vi "LeftClick.vi"(6 "Double Click":bool, 7 "Table History ref":refnum<vi>, 8 "error in (no error)":errorcluster, 9 "Table CtlRef In":refnum<vi>, 10 "Cell Position":T1, 11 "ModeCol in":refnum<class "ModeCol.lvclass">) -> (0 "error out":errorcluster, 1 "Table CtlRef Out":refnum<vi>, 2 "Discard?":bool, 3 "ModeCol out":refnum<class "ModeCol.lvclass">, 5 "Button":u16=1)   [LabVIEW 2013, in "ModeCol.lvclass"]
doc: "In the mode column, left-click should trigger a shorcut menu contining the possible modes. Right-click will bring up a different shortcut menu. Presently this column DOES modify column data (to store click button)"
uses:
  ModeCol.lvclass
  <vilib>/Utility/miscctls.llb/LVRowAndColumnTypeDef.ctl
  TypeDefs/TableHistory.ctl
  TypeDefs/TableArray.ctl
  ModeCol.lvclass/ModeCol.ctl
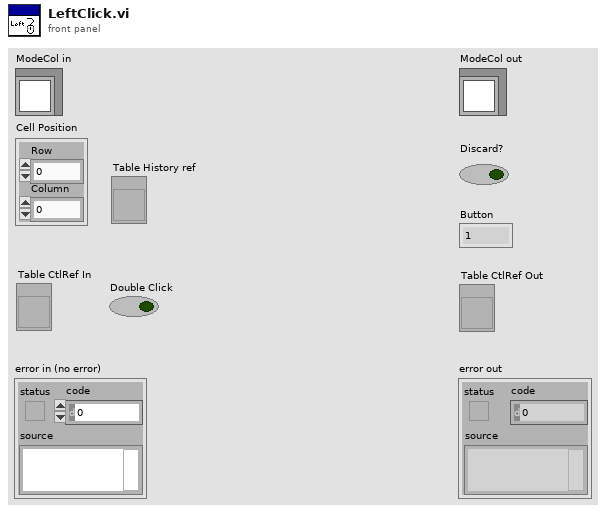
[diagram p1: front panel]
types:
  T1 = typedef "LVRowAndColumnTypeDef.ctl" = cluster{"Row":i32, "Column":i32}
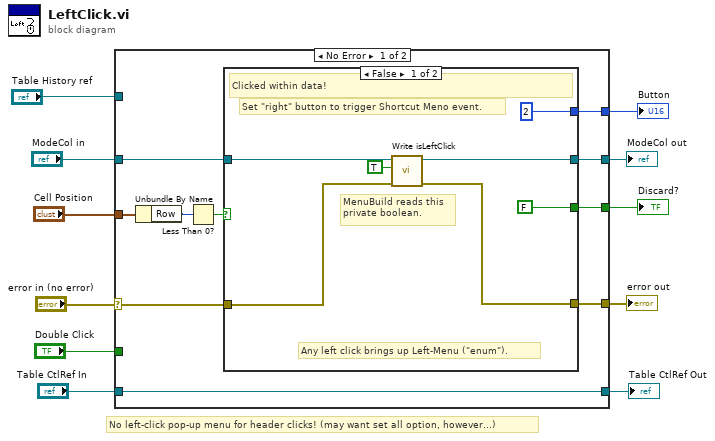
[diagram p0: block diagram]
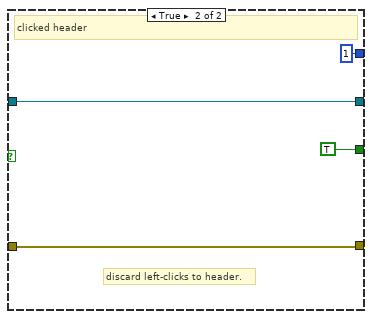
[diagram p2: hidden frame]
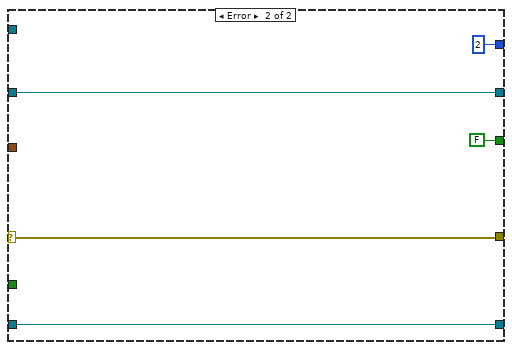
[diagram p3: hidden frame]
diagram:
  # "No left-click pop-up menu for header clicks! (may want set all option, however...)"
  n1 = case shown="No Error" "error in (no error)" {
    selector: "error in (no error)" -> [w12 w36]
    tunnel: [w21 FALSE ("Discard?")] -> w11
    tunnel: [w20 u16 2 ("Button")] -> w10
    tunnel: "ModeCol in" -> [w19 w34]
    tunnel: [w18 w34] -> w8
    tunnel: [w17 w36] -> w7
    tunnel: "Cell Position" -> [w16 _]
    tunnel: "Table History ref" -> [_ _]
    tunnel: [w13 w37] -> w5
    tunnel: "Table CtlRef In" -> [w13 w37]
    tunnel: "Double Click" -> [_ _]
    frame No Error {
      n2 = Unbundle By Name(w16) -> ("Row"=w15:i32)
      n3 = Less Than 0?(x=w15) -> (x < 0?=w14:bool)
      n4 = case shown="False" w14 {
        tunnel: [FALSE ("Discard?") TRUE ("Discard?")] -> w21
        tunnel: [u16 2 ("Button") u16 1 ("Button")] -> w20
        tunnel: w19 -> [w26 w30]
        tunnel: [w25 w30] -> w18
        tunnel: [w24 w32] -> w17
        tunnel: w12 -> [w23 w32]
        frame False {
          # "MenuBuild reads this\nprivate boolean."
          # "Set \"right\" button to trigger Shortcut Meno event."
          # "Any left click brings up Left-Menu (\"enum\")."
          # "Clicked within data!"
          n5 = call "Write isLeftClick.vi"("error in (no error)"=w23, "isLeftClick?"=TRUE ("Left Click?"), "ModeCol in"=w26) -> ("error out"=w24:errorcluster, "ModeCol out"=w25:refnum<class "ModeCol.lvclass">)  [unwired: 7 in]
        }
        frame True {
          # "discard left-clicks to header."
          # "clicked header"
        }
      }
    }
    frame Error {
    }
  }
  "error out" <- w7
  "ModeCol out" <- w8
  "Discard?" <- w11
  "Table CtlRef Out" <- w5
  "Button" <- w10
